vi "CCD Loop.vi"(8 "error in (no error)":errorcluster caption="错误输入（无错误）", 9 "数据通知器":refnum<notifier>, 10 "CAM":refnum<queue>, 11 "Director":refnum<queue>) -> (0 "error out":errorcluster caption="错误输出")   [LabVIEW 2015, in "CCD.lvlib"]
doc: "该消息循环负责处理硬件数据采集的相关消息。"
uses:
  CCD.lvlib
  <vilib>/vision/Image Controls.llb/IMAQ Image.ctl
  support/Message Queue/Message Cluster.ctl
  DAQ/Support/DAQ State.ctl
  Support/CCD Configuration.ctl
  <vilib>/userdefined/High Color/IMAQdx.ctl
  support/Message Queue/Enqueue Message (Single).vi
  <vilib>/Utility/error.llb/Error Cluster From Error Code.vi
  <vilib>/ErrorRing/Error Ring.xnode
  support/Message Queue/Message Queue.lvlib
  DAQ/DAQ.lvlib
  <vilib>/vision/driver/NI_Vision_Acquisition_Software.lvlib
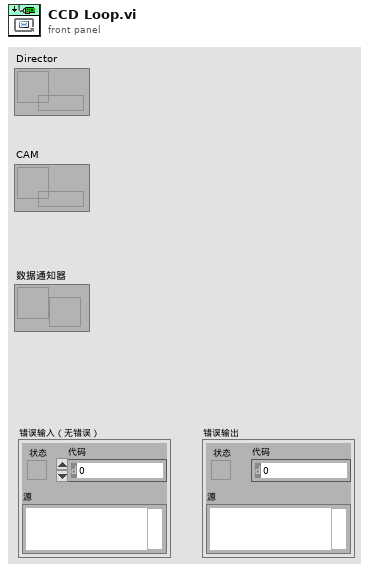
[diagram p1: front panel]
types:
  T1 = typedef "CCD.lvlib/CCD Configuration.ctl" = cluster{"Session In":T2, "New Image":T3}
  T2 = typedef "IMAQdx.ctl" = refnum<k21>
  T3 = typedef "IMAQ Image.ctl" = refnum<image>
  T4 = typedef "DAQ.lvlib/DAQ State.ctl" = enum16{"Idle", "Acquiring"}
  T5 = typedef "Image Type" = u32
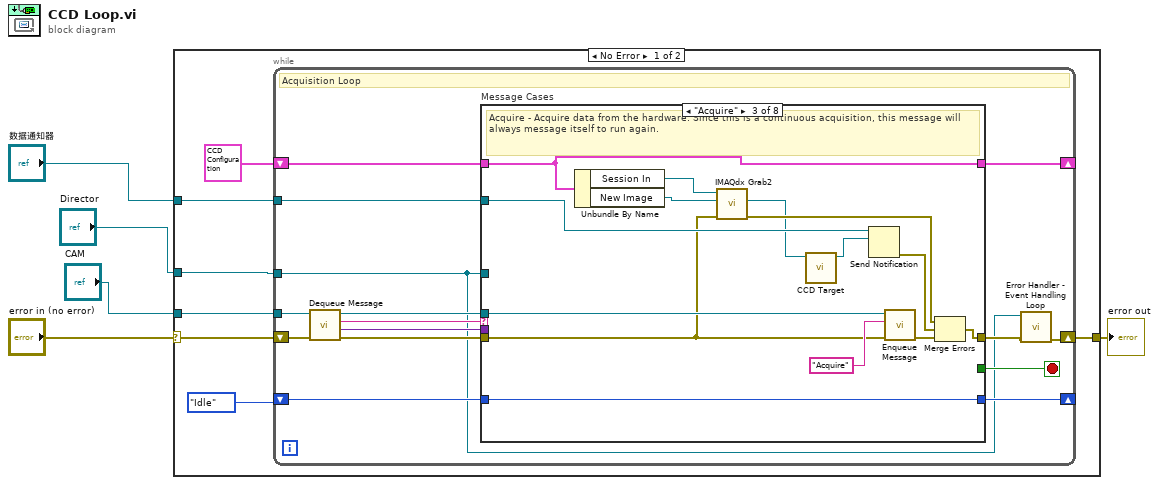
[diagram p0: block diagram]
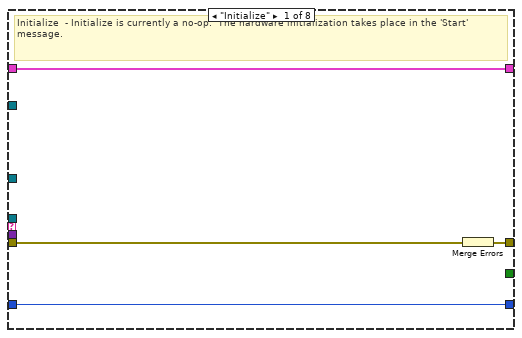
[diagram p2: hidden frame]
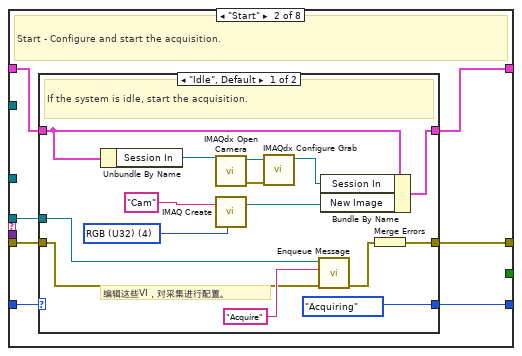
[diagram p3: hidden frame]
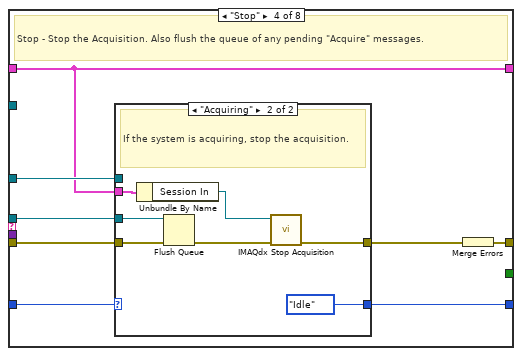
[diagram p5: hidden frame]
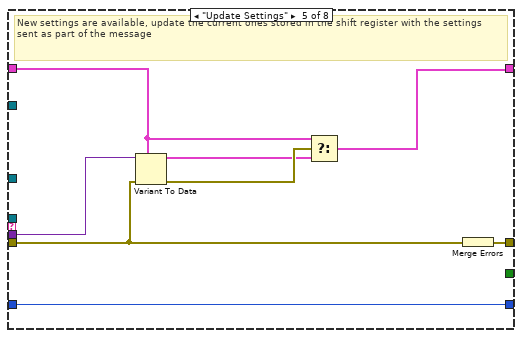
[diagram p7: hidden frame]
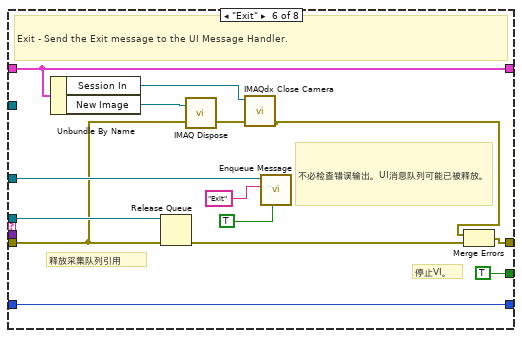
[diagram p8: hidden frame]
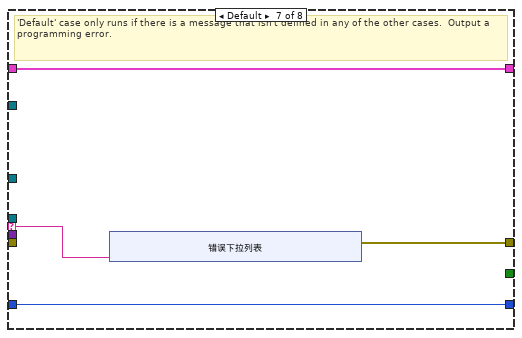
[diagram p9: hidden frame]
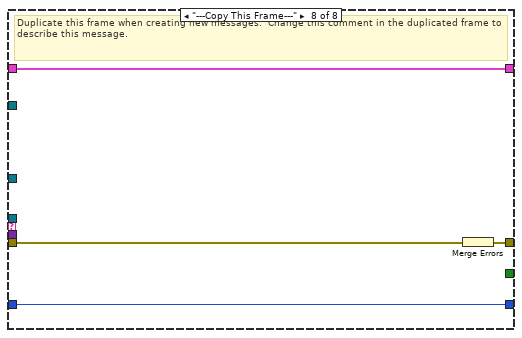
[diagram p10: hidden frame]
diagram:
  n1 = case shown="No Error" "error in (no error)" {
    selector: "error in (no error)" -> [w11 w125]
    tunnel: [w12 w125] -> w5
    tunnel: "数据通知器" -> [w9 _]
    tunnel: "CAM" -> [w8 _]
    tunnel: "Director" -> [w7 _]
    frame No Error {
      n2 = while {
        tunnel: w8 -> [w19]
        shift-right: [w26] -> _
        shift-left: T1 {"Session In"="", "New Image"=refnum} ("CCD Configuration") -> [w27]
        shift-right: [w16] -> w12
        shift-left: w11 -> [w24]
        tunnel: w7 -> [w14]
        shift-right: [w17] -> _
        shift-left: DAQ_State."Idle" ("State") -> [w18]
        tunnel: w9 -> [w13]
        stop <- w25 stop-if-true
        # "Acquisition Loop"
        n3 = call "Dequeue Message.vi"("error in (no error)"=w24, "消息队列"=w19) -> ("error out"=w23:cluster{"状态":bool, "代码":i32, "源":string}, "消息数据"=w21:variant, "消息"=w22:string, "消息队列副本"=w20:refnum<queue>)  [unwired: 6 in]
        n4 = case "Message Cases" shown="\"Acquire\"" w22 {
          selector: w22 -> [_ _ _ _ _ _ w112 _]
          tunnel: w20 -> [_ w35 w68 w76 _ w103 _ _]
          tunnel: w23 -> [w29 w36 w63 w77 w89 w99 _ w124]
          tunnel: [w31 w38 w70 w78 w95 w108 w111 w122] -> w15
          tunnel: w27 -> [w28 w37 w61 w71 w91 w101 w113 w123]
          tunnel: [w28 w34 w61 w71 w90 w101 w113 w123] -> w26
          tunnel: [_ _ _ _ _ TRUE _ _] -> w25
          tunnel: w21 -> [_ _ _ _ w94 _ _ _]
          tunnel: w14 -> [_ _ _ w75 _ w107 _ _]
          tunnel: w18 -> [w30 w33 w66 w74 w88 w102 w110 w121]
          tunnel: [w30 w32 w66 w73 w88 w102 w110 w121] -> w17
          tunnel: w13 -> [_ _ w65 _ _ _ _ _]
          frame "Initialize" {
            # "Initialize  - Initialize is currently a no-op.  The hardware initialization takes place in the 'Start' message."
            n5 = Merge Errors(w29) -> (w31:errorcluster)
          }
          frame "Start" {
            # "Start - Configure and start the acquisition."
            n6 = case shown="\"Idle\", Default" w33 {
              selector: w33 -> [_ w54]
              tunnel: [w53 w56] -> w38
              tunnel: w37 -> [w42 w55]
              tunnel: w36 -> [w48 w56]
              tunnel: w35 -> [w51 _]
              tunnel: [w40 w55] -> w34
              tunnel: [DAQ_State."Acquiring" ("State") w54] -> w32
              frame "Idle", Default {
                w43 = T5 4 items=["Grayscale (U8)", "Grayscale (I16)", "Grayscale (SGL)", "Complex (CSG)", "RGB (U32)", "HSL (U32)", "RGB (U64)", "Grayscale (U16)"] ("Image Type")
                # "编辑这些VI，对采集进行配置。"
                # "If the system is idle, start the acquisition."
                n7 = Unbundle By Name(w42) -> ("Session In"=w45:T2)
                n8 = call <vilib>:"IMAQdx Open Camera.vi"("Session In"=w45) -> ("error out"=w47:errorcluster, "Session Out"=w46:T2)  [unwired: 9 in]
                n9 = call "IMAQ Create"("Image Name"="Cam", "Image Type"=w43) -> ("New Image"=w41:T3)  [unwired: 3 in, 1 out]
                n10 = call <vilib>:"IMAQdx Configure Grab.vi"("error in"=w47, "Session In"=w46) -> ("Session Out"=w39:T2)  [unwired: 8 in, 1 out]
                n11 = call-poly "Enqueue Message.vi"("error in (no error)"=w48, "消息"="Acquire" ("Message"), "消息队列"=w51) -> ("error out"=w52:cluster{"状态":bool, "代码":i32, "源":string})  [unwired: 7 in, 1 out]
                n12 = Bundle By Name(cluster=w42, "Session In"=w39, "New Image"=w41) -> (w40:T1)
                n13 = Merge Errors(w52) -> (w53:errorcluster)
              }
              frame "Acquiring" {
                # "The system is already acquiring. Ignore the \"Start\" message."
              }
            }
          }
          frame "Acquire" {
            # "Acquire - Acquire data from the hardware. Since this is a continuous acquisition, this message will always message itself to run again."
            n14 = Unbundle By Name(w61) -> ("Session In"=w60:T2, "New Image"=w59:T3)
            n15 = call <vilib>:"IMAQdx Grab2.vi"("error in"=w63, "Image In"=w59, "Session In"=w60) -> ("error out"=w62:errorcluster, "Image Out"=w58:T3)  [unwired: 5 in, 2 out]
            n16 = call "CCD Target.vi"("Image"=w58) -> ("Image Out"=w57:T3)  [unwired: 9 in, 1 out]
            n17 = Send Notification(notification=w57, notifier=w65) -> (error out=w64:errorcluster)  [unwired: 1 in, 1 out]
            n18 = call-poly "Enqueue Message.vi"("error in (no error)"=w63, "消息"="Acquire" ("Message"), "消息队列"=w68) -> ("error out"=w69:cluster{"状态":bool, "代码":i32, "源":string})  [unwired: 7 in, 1 out]
            n19 = Merge Errors(w62, w64, w69) -> (w70:errorcluster)
          }
          frame "Stop" {
            # "Stop - Stop the Acquisition. Also flush the queue of any pending \"Acquire\" messages."
            n20 = case shown="\"Acquiring\"" w74 {
              selector: w74 -> [w80 _]
              tunnel: w77 -> [w79 w87]
              tunnel: w76 -> [_ w86]
              tunnel: w75 -> [_ _]
              tunnel: [w80 DAQ_State."Idle" ("State")] -> w73
              tunnel: [w79 w83] -> w72
              tunnel: w71 -> [_ w82]
              frame "Idle", Default {
                # "The system is already idle. Ignore the \"Stop\" message."
              }
              frame "Acquiring" {
                # "If the system is acquiring, stop the acquisition."
                n21 = Unbundle By Name(w82) -> ("Session In"=w81:T2)
                n22 = Flush Queue(queue=w86, error in (no error)=w87) -> (error out=w84:errorcluster)  [unwired: 2 out]
                n23 = call <vilib>:"IMAQdx Stop Acquisition.vi"("error in"=w84, "Session In"=w81) -> ("error out"=w83:errorcluster)  [unwired: 8 in, 1 out]
              }
            }
            n24 = Merge Errors(w72) -> (w78:errorcluster)
          }
          frame "Update Settings" {
            # "New settings are available, update the current ones stored in the shift register with the settings sent as part of the message"
            n25 = Variant To Data(error in=w89, type=w91, Variant=w94) -> (data=w92:T1, error out=w93:errorcluster)
            n26 = Select(t=w91, s=w93, f=w92) -> (s? t:f=w90:T1)
            n27 = Merge Errors(w89) -> (w95:errorcluster)
          }
          frame "Exit" {
            # "不必检查错误输出。UI消息队列可能已被释放。"
            # "释放采集队列引用"
            # "停止VI。"
            # "Exit - Send the Exit message to the UI Message Handler."
            n28 = Unbundle By Name(w101) -> ("Session In"=w96:T2, "New Image"=w97:T3)
            n29 = Release Queue(queue=w103, error in (no error)=w99) -> (error out=w104:errorcluster)  [unwired: 1 in, 2 out]
            n30 = call "IMAQ Dispose"("Image"=w97, "error in (no error)"=w99) -> ("error out"=w100:errorcluster)  [unwired: 4 in]
            n31 = call <vilib>:"IMAQdx Close Camera.vi"("error in"=w100, "Session In"=w96) -> ("error out"=w98:errorcluster)  [unwired: 9 in]
            n32 = call-poly "Enqueue Message.vi"("优先消息？ (F)"=TRUE, "消息"="Exit" ("Message"), "消息队列"=w107) -> ()  [unwired: 7 in, 2 out]
            n33 = Merge Errors(w98, w104) -> (w108:errorcluster)
          }
          frame Default {
            # "'Default' case only runs if there is a message that isn't defined in any of the other cases.  Output a programming error."
            n34 = xnode "错误下拉列表"("parameter 0"=w112) -> ("error out"=w111:errorcluster)
          }
          frame "---Copy This Frame---" {
            # "Duplicate this frame when creating new messages.  Change this comment in the duplicated frame to describe this message."
            n35 = Merge Errors(w124) -> (w122:errorcluster)
          }
        }
        n36 = call "Error Handler - Event Handling Loop.vi"("error in (no error)"=w15, "消息队列"=w14) -> ("错误输入副本"=w16:cluster{"状态":bool, "代码":i32, "源":string})  [unwired: 8 in, 1 out]
      }
    }
    frame Error {
    }
  }
  "error out" <- w5
